vi "pressure min.vi"(0 "unsigned byte array":u8[](array[numeric])) -> (10 "x-y 9":dbl, 11 "x-y 10":dbl, 12 "x-y 7":dbl, 13 "x-y 8":dbl, 14 "x-y 1":dbl, 15 "x-y 2":dbl, 16 "x-y 3":dbl, 17 "x-y 4":dbl, 18 "x-y 5":dbl, 19 "x-y 6":dbl)   [LabVIEW 2016]
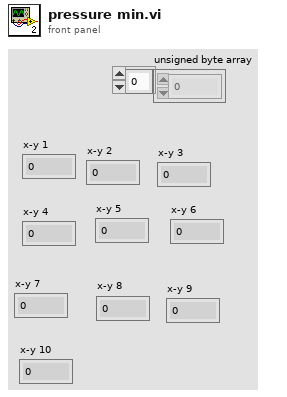
[diagram p1: front panel]
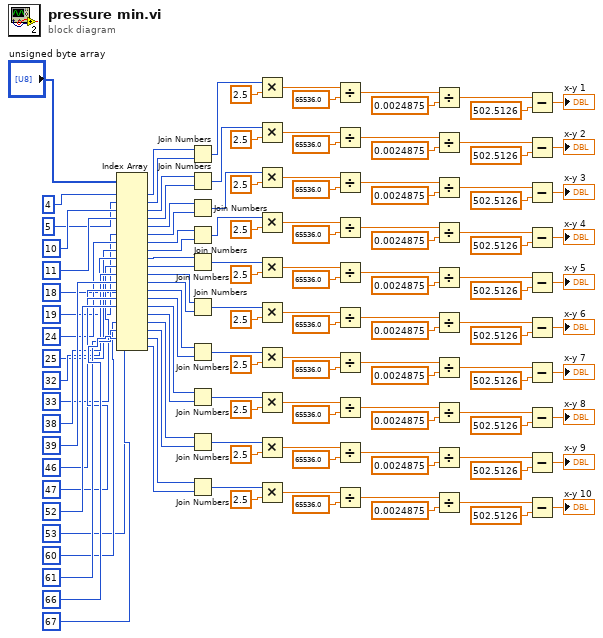
[diagram p0: block diagram]
diagram:
  n1 = Index Array(array="unsigned byte array", index #1=4 ("index"), index #2=5 ("index"), index #3=10 ("index"), index #4=11 ("index"), index #5=18 ("index"), index #6=19 ("index"), index #7=24 ("index"), index #8=25 ("index"), index #9=32 ("index"), index #10=33 ("index"), index #11=38 ("index"), index #12=39 ("index"), index #13=46 ("index"), index #14=47 ("index"), index #15=52 ("index"), index #16=53 ("index"), index #17=60 ("index"), index #18=61 ("index"), index #19=66 ("index"), index #20=67 ("index")) -> (element #1=w90:u8, element #2=w89:u8, element #3=w16:u8, element #4=w15:u8, element #5=w14:u8, element #6=w13:u8, element #7=w12:u8, element #8=w11:u8, element #9=w10:u8, element #10=w9:u8, element #11=w8:u8, element #12=w7:u8, element #13=w6:u8, element #14=w5:u8, element #15=w4:u8, element #16=w3:u8, element #17=w2:u8, element #18=w1:u8, element #19=w101:u8, element #20=w100:u8)
  n2 = Join Numbers(hi=w90, lo=w89) -> ((hi.lo)=w92:u16)
  n3 = Join Numbers(hi=w16, lo=w15) -> ((hi.lo)=w81:u16)
  n4 = Join Numbers(hi=w14, lo=w13) -> ((hi.lo)=w72:u16)
  n5 = Join Numbers(hi=w12, lo=w11) -> ((hi.lo)=w63:u16)
  n6 = Join Numbers(hi=w10, lo=w9) -> ((hi.lo)=w54:u16)
  n7 = Join Numbers(hi=w8, lo=w7) -> ((hi.lo)=w45:u16)
  n8 = Join Numbers(hi=w6, lo=w5) -> ((hi.lo)=w36:u16)
  n9 = Join Numbers(hi=w4, lo=w3) -> ((hi.lo)=w27:u16)
  n10 = Join Numbers(hi=w2, lo=w1) -> ((hi.lo)=w18:u16)
  n11 = Join Numbers(hi=w101, lo=w100) -> ((hi.lo)=w103:u16)
  n12 = Multiply(x=w92, y=2.5) -> (x*y=w98:dbl)
  n13 = Multiply(x=w81, y=2.5) -> (x*y=w87:dbl)
  n14 = Multiply(x=w72, y=2.5) -> (x*y=w78:dbl)
  n15 = Multiply(x=w63, y=2.5) -> (x*y=w69:dbl)
  n16 = Multiply(x=w54, y=2.5) -> (x*y=w60:dbl)
  n17 = Multiply(x=w45, y=2.5) -> (x*y=w51:dbl)
  n18 = Multiply(x=w36, y=2.5) -> (x*y=w42:dbl)
  n19 = Multiply(x=w27, y=2.5) -> (x*y=w33:dbl)
  n20 = Multiply(x=w18, y=2.5) -> (x*y=w24:dbl)
  n21 = Multiply(x=w103, y=2.5) -> (x*y=w109:dbl)
  n22 = Divide(x=w98, y=65536.0) -> (x/y=w96:dbl)
  n23 = Divide(x=w87, y=65536.0) -> (x/y=w85:dbl)
  n24 = Divide(x=w78, y=65536.0) -> (x/y=w76:dbl)
  n25 = Divide(x=w69, y=65536.0) -> (x/y=w67:dbl)
  n26 = Divide(x=w60, y=65536.0) -> (x/y=w58:dbl)
  n27 = Divide(x=w51, y=65536.0) -> (x/y=w49:dbl)
  n28 = Divide(x=w42, y=65536.0) -> (x/y=w40:dbl)
  n29 = Divide(x=w33, y=65536.0) -> (x/y=w31:dbl)
  n30 = Divide(x=w24, y=65536.0) -> (x/y=w22:dbl)
  n31 = Divide(x=w109, y=65536.0) -> (x/y=w107:dbl)
  n32 = Divide(x=w96, y=0.0024875) -> (x/y=w99:dbl)
  n33 = Divide(x=w85, y=0.0024875) -> (x/y=w88:dbl)
  n34 = Divide(x=w76, y=0.0024875) -> (x/y=w79:dbl)
  n35 = Divide(x=w67, y=0.0024875) -> (x/y=w70:dbl)
  n36 = Divide(x=w58, y=0.0024875) -> (x/y=w61:dbl)
  n37 = Divide(x=w49, y=0.0024875) -> (x/y=w52:dbl)
  n38 = Divide(x=w40, y=0.0024875) -> (x/y=w43:dbl)
  n39 = Divide(x=w31, y=0.0024875) -> (x/y=w34:dbl)
  n40 = Divide(x=w22, y=0.0024875) -> (x/y=w25:dbl)
  n41 = Divide(x=w107, y=0.0024875) -> (x/y=w110:dbl)
  n42 = Subtract(x=w99, y=502.5126) -> (x-y=→"x-y 1":dbl)
  n43 = Subtract(x=w88, y=502.5126) -> (x-y=→"x-y 2":dbl)
  n44 = Subtract(x=w79, y=502.5126) -> (x-y=→"x-y 3":dbl)
  n45 = Subtract(x=w70, y=502.5126) -> (x-y=→"x-y 4":dbl)
  n46 = Subtract(x=w61, y=502.5126) -> (x-y=→"x-y 5":dbl)
  n47 = Subtract(x=w52, y=502.5126) -> (x-y=→"x-y 6":dbl)
  n48 = Subtract(x=w43, y=502.5126) -> (x-y=→"x-y 7":dbl)
  n49 = Subtract(x=w34, y=502.5126) -> (x-y=→"x-y 8":dbl)
  n50 = Subtract(x=w25, y=502.5126) -> (x-y=→"x-y 9":dbl)
  n51 = Subtract(x=w110, y=502.5126) -> (x-y=→"x-y 10":dbl)
